vi "Write Tree Refnum.vi"(8 "error in":errorcluster, 10 "Tree Refnum":refnum<vi>, 11 "Report Viewer in":refnum<class "Report Viewer.lvclass">) -> (0 "error out":errorcluster, 3 "Report Viewer out":refnum<class "Report Viewer.lvclass">)   [LabVIEW 2023, in "Report Viewer.lvlib" / "Report Viewer.lvclass"]
uses:
  Library/Report Viewer.lvclass
  Library/Report Viewer.lvclass/Report Viewer.ctl
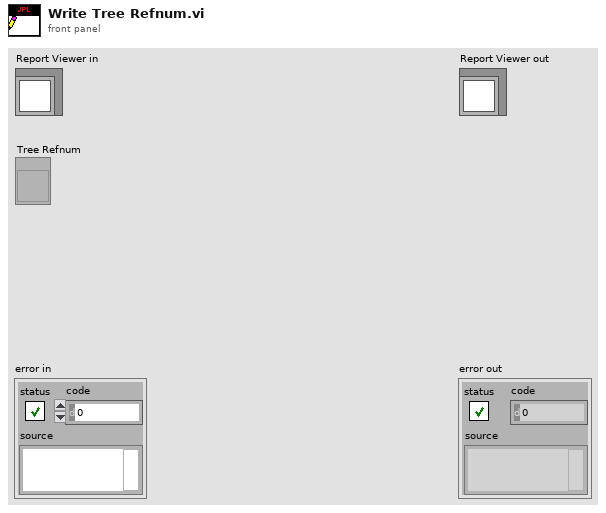
[diagram p1: front panel]
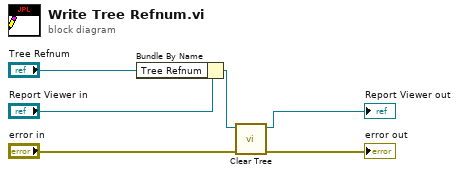
[diagram p0: block diagram]
diagram:
  n1 = Bundle By Name(cluster="Report Viewer in", "Tree Refnum"="Tree Refnum") -> (w4:refnum<class "Report Viewer.lvclass">)
  n2 = call "Clear Tree.vi"("error in"="error in", "Report Viewer in"=w4) -> ("error out"=→"error out":errorcluster, "Report Viewer out"=→"Report Viewer out":refnum<class "Report Viewer.lvclass">)  [unwired: 8 in]
